vi "Untitled 1 (2).vi"() -> ()   [LabVIEW 2013]
panel:
  out "Waveform Chart":dynamicdata(graph)
  out "Boolean 7":bool
  out "Boolean 6":bool
  out "Boolean 5":bool
  out "Boolean 4":bool
  out "Boolean 3":bool
  out "Boolean 2":bool
  in  "Triangle":bool
  in  "Random":bool
  in  "Arbitary":bool
  in  "Sine":bool
  in  "Square":bool
  in  "Sawtooth":bool
  in  "stop":bool
  in  "Phase":dbl
  in  "Amplitude":dbl=10.0
  in  "Frequency":dbl=10.1
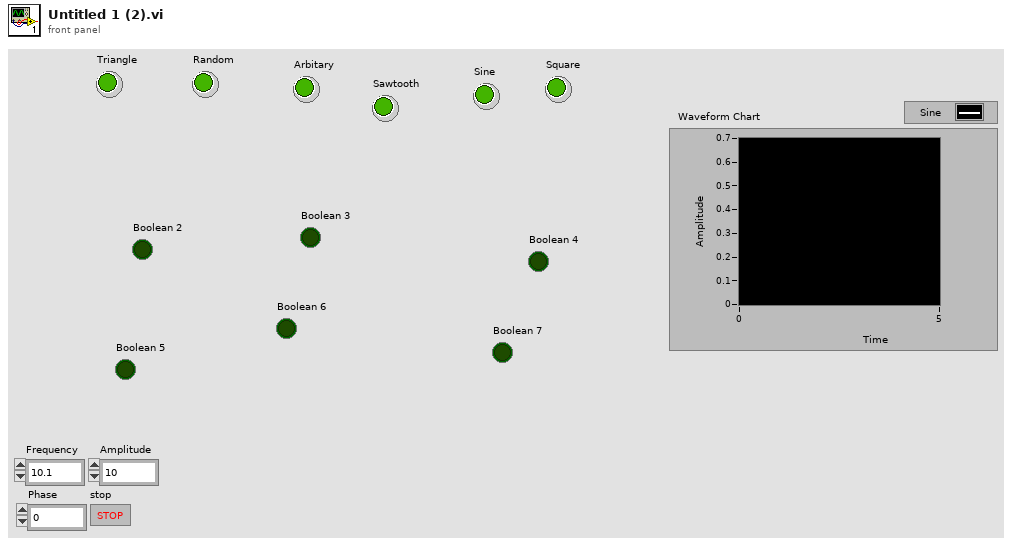
[diagram p1: front panel]
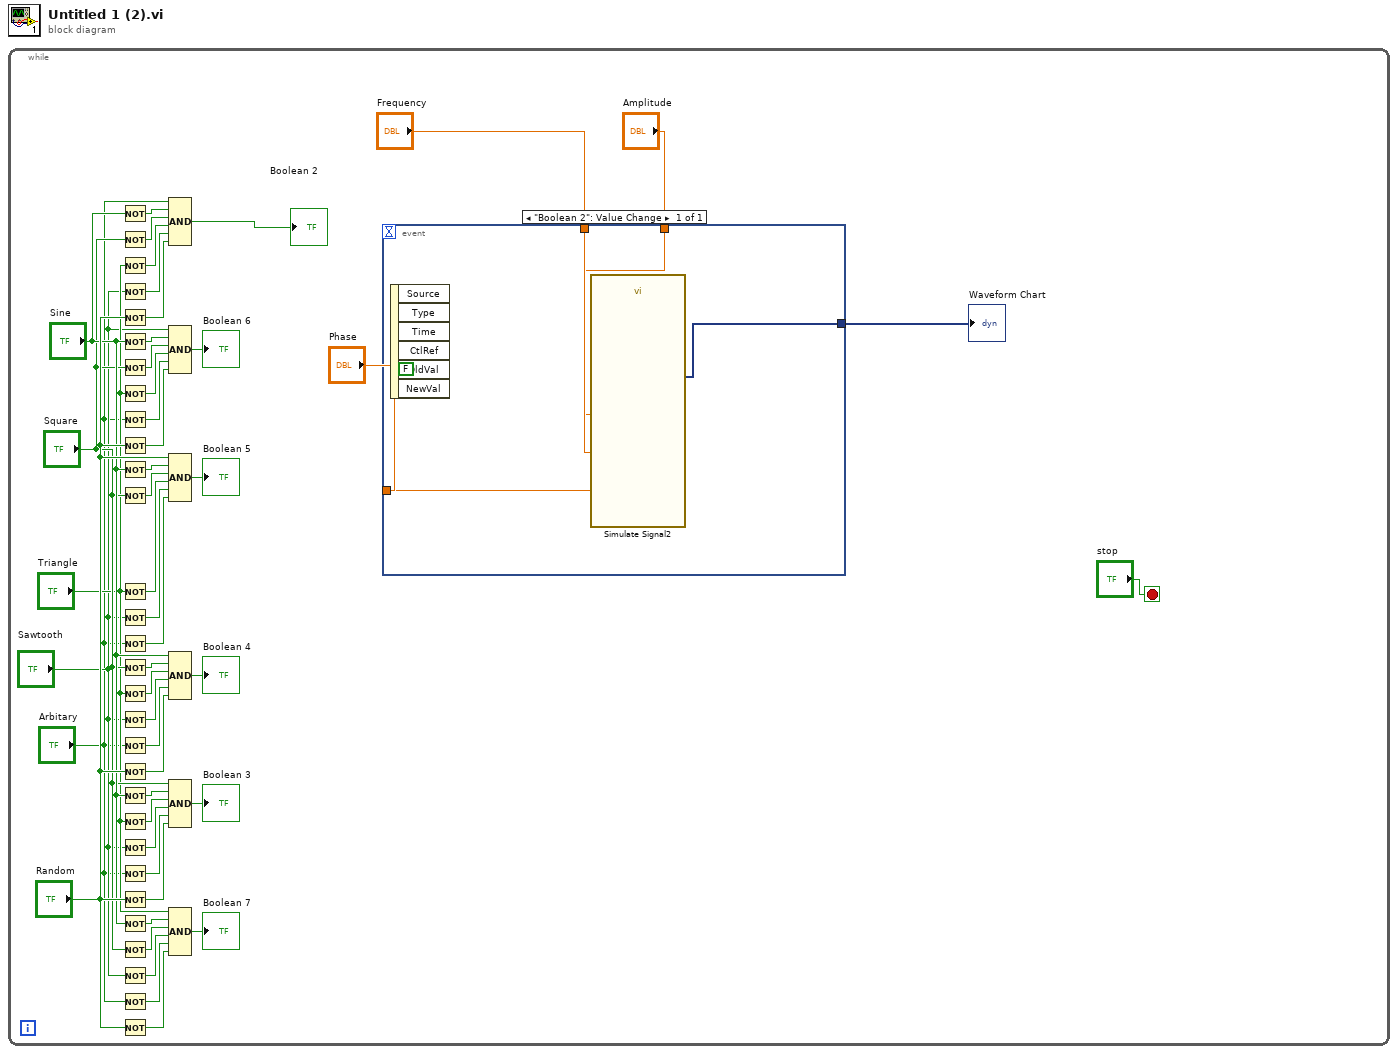
[diagram p0: block diagram]
diagram:
  n1 = while {
    stop <- "stop" stop-if-true
    n2 = Not(x="Sine") -> (.not. x?=w26:bool)
    n3 = Not(x="Square") -> (.not. x?=w25:bool)
    n4 = Not(x="Triangle") -> (.not. x?=w24:bool)
    n5 = Not(x="Sawtooth") -> (.not. x?=w23:bool)
    n6 = Not(x="Random") -> (.not. x?=w22:bool)
    n7 = Not(x="Sine") -> (.not. x?=w31:bool)
    n8 = Not(x="Square") -> (.not. x?=w30:bool)
    n9 = Not(x="Triangle") -> (.not. x?=w29:bool)
    n10 = Not(x="Arbitary") -> (.not. x?=w28:bool)
    n11 = Not(x="Random") -> (.not. x?=w27:bool)
    n12 = Not(x="Sine") -> (.not. x?=w21:bool)
    n13 = Not(x="Square") -> (.not. x?=w20:bool)
    n14 = Not(x="Triangle") -> (.not. x?=w19:bool)
    n15 = Not(x="Sawtooth") -> (.not. x?=w18:bool)
    n16 = Not(x="Arbitary") -> (.not. x?=w17:bool)
    n17 = Not(x="Square") -> (.not. x?=w46:bool)
    n18 = Not(x="Triangle") -> (.not. x?=w45:bool)
    n19 = Not(x="Sawtooth") -> (.not. x?=w44:bool)
    n20 = Not(x="Arbitary") -> (.not. x?=w43:bool)
    n21 = Not(x="Random") -> (.not. x?=w42:bool)
    n22 = Not(x="Sine") -> (.not. x?=w41:bool)
    n23 = Not(x="Triangle") -> (.not. x?=w40:bool)
    n24 = Not(x="Sawtooth") -> (.not. x?=w39:bool)
    n25 = Not(x="Arbitary") -> (.not. x?=w38:bool)
    n26 = Not(x="Random") -> (.not. x?=w37:bool)
    n27 = Not(x="Sine") -> (.not. x?=w36:bool)
    n28 = Not(x="Square") -> (.not. x?=w35:bool)
    n29 = Not(x="Sawtooth") -> (.not. x?=w34:bool)
    n30 = Not(x="Arbitary") -> (.not. x?=w33:bool)
    n31 = Not(x="Random") -> (.not. x?=w32:bool)
    n32 = Compound Arithmetic op=AND("Arbitary", w26, w25, w24, w23, w22) -> (→"Boolean 2":bool)
    n33 = Compound Arithmetic op=AND("Sawtooth", w31, w30, w29, w28, w27) -> (→"Boolean 6":bool)
    n34 = Compound Arithmetic op=AND("Random", w21, w20, w19, w18, w17) -> (→"Boolean 5":bool)
    n35 = Compound Arithmetic op=AND("Sine", w46, w45, w44, w43, w42) -> (→"Boolean 4":bool)
    n36 = Compound Arithmetic op=AND("Square", w41, w40, w39, w38, w37) -> (→"Boolean 3":bool)
    n37 = Compound Arithmetic op=AND("Triangle", w36, w35, w34, w33, w32) -> (→"Boolean 7":bool)
    n38 = event shown="[0] \"Boolean 2\": Value Change" {
      selector: _ -> [_]
      dyn-events: _ -> [_]
      timeout: _ -> [_]
      tunnel: [w51] -> w4
      tunnel: "Frequency" -> [w50]
      tunnel: "Amplitude" -> [w49]
      tunnel: "Phase" -> [w48]
      event "Boolean 2": Value Change {
        (unwired) FALSE ("OldVal")
        n39 = event-data() -> ()  [unwired: 1 in, 6 out]
        n40 = call "Simulate Signal2"("Frequency"=w50, "Amplitude"=w49, "Phase"=w48) -> ("Sine"=w51:dynamicdata)  [unwired: 11 in, 1 out]
      }
    }
    "Waveform Chart" <- w4
  }
